vi "统一指令集.vi"(8 "Error In":errorcluster caption="错误输入", 10 "设置参数":string, 11 "统一指令集":T1=enum."波特率切换为9600") -> (0 "Error Out":errorcluster caption="错误输出", 2 "应答":string, 3 "指令":string)   [LabVIEW 2020]
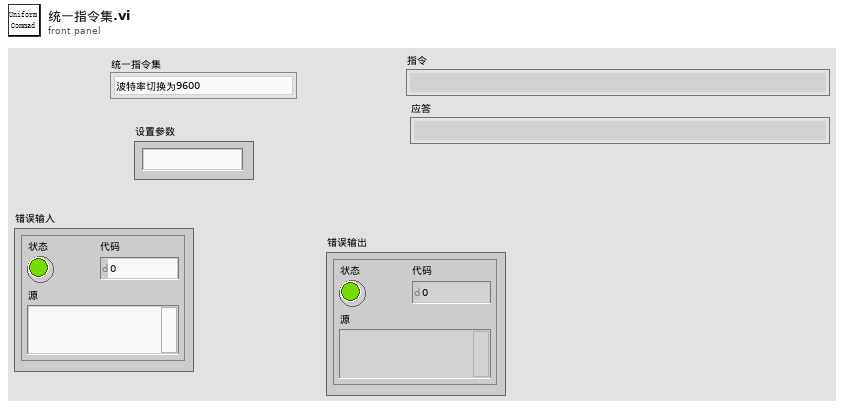
[diagram p1: front panel]
types:
  T1 = typedef "统一指令集.ctl" = enum16{"无操作", "自定义", "波特率切换为9600", "波特率切换为115200", "拍图/解码", "取图", "电平触发模式", "连续读码模式", "睡眠模式", "获取图像分辨率", "开启RTS与CTS流控", "无流控", "感应模式", "红外感应模式", "图像感应模式", "图像与红外感应模式", "切换为串口", "切换为CDC", "关闭照明灯", "开启照明灯", "照明灯常亮", "关闭瞄准灯", "开启瞄准灯", "开启设置码", "连续读码模式2", "触发模式", "0390命令识读模式", "0390连续识读模式", "查询产品序列号", "查询SN空间大小", "产品信息修改开关", "设置产品序列号", "删除序列号", "0390单芯片开启EEPROM写入", "0390单芯片关闭EEPROM写入", "0390单芯片写入产品序列号", "0390单芯片查询产品序列号"}
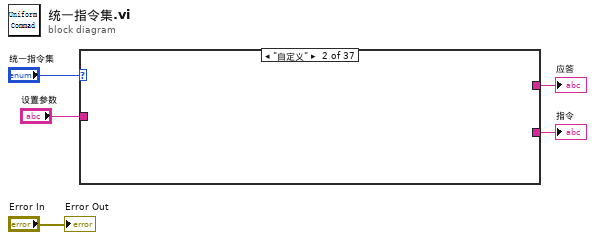
[diagram p0: block diagram]
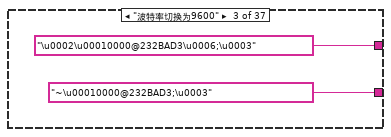
[diagram p3: hidden frame]
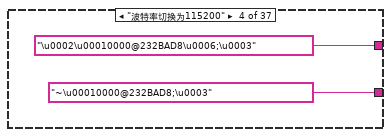
[diagram p4: hidden frame]
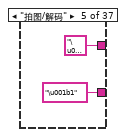
[diagram p5: hidden frame]
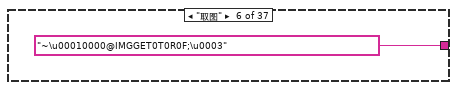
[diagram p6: hidden frame]
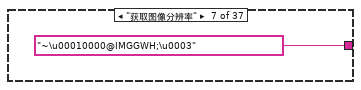
[diagram p7: hidden frame]
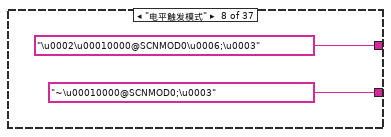
[diagram p8: hidden frame]
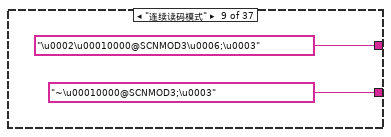
[diagram p9: hidden frame]
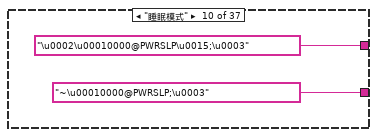
[diagram p10: hidden frame]
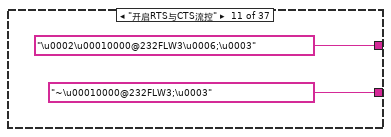
[diagram p11: hidden frame]
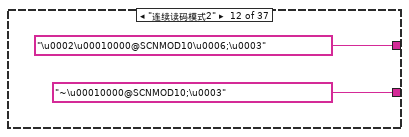
[diagram p12: hidden frame]
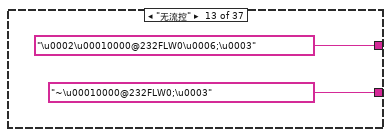
[diagram p13: hidden frame]
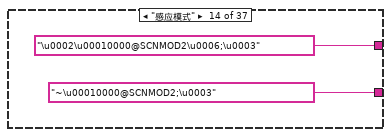
[diagram p14: hidden frame]
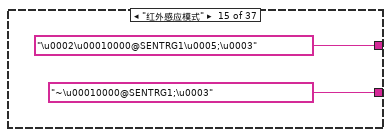
[diagram p15: hidden frame]
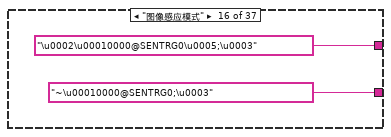
[diagram p16: hidden frame]
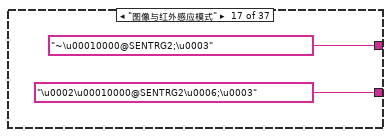
[diagram p17: hidden frame]
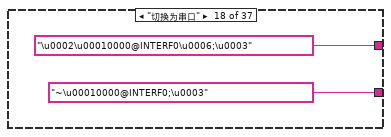
[diagram p18: hidden frame]
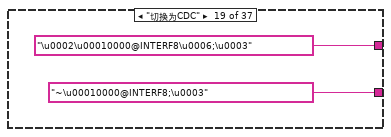
[diagram p19: hidden frame]
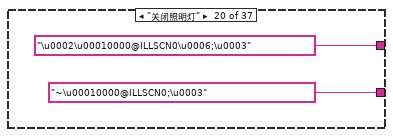
[diagram p20: hidden frame]
diagram:
  n1 = case shown="\"自定义\"" "统一指令集" {
    tunnel: [_ _ "~\u00010000@232BAD3;\u0003" "~\u00010000@232BAD8;\u0003" "\u001b1" "~\u00010000@IMGGET0T0R0F;\u0003" "~\u00010000@IMGGWH;\u0003" "~\u00010000@SCNMOD0;\u0003" "~\u00010000@SCNMOD3;\u0003" "~\u00010000@PWRSLP;\u0003" "~\u00010000@232FLW3;\u0003" "~\u00010000@SCNMOD10;\u0003" "~\u00010000@232FLW0;\u0003" "~\u00010000@SCNMOD2;\u0003" "~\u00010000@SENTRG1;\u0003" "~\u00010000@SENTRG0;\u0003" "\u0002\u00010000@SENTRG2\u0006;\u0003" "~\u00010000@INTERF0;\u0003" "~\u00010000@INTERF8;\u0003" "~\u00010000@ILLSCN0;\u0003" "~\u00010000@ILLSCN1;\u0003" "~\u00010000@ILLSCN2;\u0003" ("设置参数") "~\u00010000@AMLENA0;\u0003" "~\u00010000@AMLENA1;\u0003" "~\u00010000@SETUPN1;\u0003" "~\u00010000@SCNMOD1;\u0003" "~\u0000\b\u0001\u0000\u0000诊\u0004" "~\u0000\b\u0001\u0000\u0000诌\"" "~\u00010000@QRYPSN;\u0003" "~\u00010000@PSNQSZ;\u0003" "~\u00010000@PINFEN1;\u0003" w65 "~\u00010000@PSNDEL;\u0003" "~\u0000\u0003\u0001\u0000\u0000\u0000˜f" "~\u0000\u0000\u0001\u0000\u0000\u0000v´" w74 "~\u0000\u0005\u0001\u0001\u0000\u0000bÓ" ("设置参数")] -> w1
    tunnel: [_ _ "\u0002\u00010000@232BAD3\u0006;\u0003" "\u0002\u00010000@232BAD8\u0006;\u0003" "\u0006" _ _ "\u0002\u00010000@SCNMOD0\u0006;\u0003" "\u0002\u00010000@SCNMOD3\u0006;\u0003" "\u0002\u00010000@PWRSLP\u0015;\u0003" "\u0002\u00010000@232FLW3\u0006;\u0003" "\u0002\u00010000@SCNMOD10\u0006;\u0003" "\u0002\u00010000@232FLW0\u0006;\u0003" "\u0002\u00010000@SCNMOD2\u0006;\u0003" "\u0002\u00010000@SENTRG1\u0005;\u0003" "\u0002\u00010000@SENTRG0\u0005;\u0003" "~\u00010000@SENTRG2;\u0003" "\u0002\u00010000@INTERF0\u0006;\u0003" "\u0002\u00010000@INTERF8\u0006;\u0003" "\u0002\u00010000@ILLSCN0\u0006;\u0003" "\u0002\u00010000@ILLSCN1\u0006;\u0003" "\u0002\u00010000@ILLSCN2\u0006;\u0003" "\u0002\u00010000@AMLENA0\u0006;\u0003" "\u0002\u00010000@AMLENA1\u0006;\u0003" "\u0002\u00010000@SETUPN1\u0006;\u0003" "\u0002\u00010000@SCNMOD1\u0006;\u0003" "\u0002\u0000\u0000\u0001\u000031" "\u0002\u0000\u0000\u0001\u000031" "\r\n\u0006;\u0003" _ "\u0002\u00010000@PINFEN1\u0006;\u0003" w62 "\u0002\u00010000@PSNDEL\u0006;\u0003" "\u0002\u0000\u0000\u0001\u000031" "\u0002\u0000\u0000\u0001\u000031" "\u0002\u0000\u0000\u0001\u000031" _] -> w4
    tunnel: "设置参数" -> [_ _ _ _ _ _ _ _ _ _ _ _ _ _ _ _ _ _ _ _ _ _ _ _ _ _ _ _ _ _ _ w61 _ _ _ w74 _]
    frame "无操作", Default {
    }
    frame "自定义" {
    }
    frame "波特率切换为9600" {
    }
    frame "波特率切换为115200" {
    }
    frame "拍图/解码" {
    }
    frame "取图" {
    }
    frame "获取图像分辨率" {
    }
    frame "电平触发模式" {
    }
    frame "连续读码模式" {
    }
    frame "睡眠模式" {
    }
    frame "开启RTS与CTS流控" {
    }
    frame "连续读码模式2" {
    }
    frame "无流控" {
    }
    frame "感应模式" {
    }
    frame "红外感应模式" {
    }
    frame "图像感应模式" {
    }
    frame "图像与红外感应模式" {
    }
    frame "切换为串口" {
    }
    frame "切换为CDC" {
    }
    frame "关闭照明灯" {
    }
    frame "开启照明灯" {
    }
    frame "照明灯常亮" {
    }
    frame "关闭瞄准灯" {
    }
    frame "开启瞄准灯" {
    }
    frame "开启设置码" {
    }
    frame "触发模式" {
    }
    frame "0390命令识读模式" {
    }
    frame "0390连续识读模式" {
    }
    frame "查询产品序列号" {
    }
    frame "查询SN空间大小" {
    }
    frame "产品信息修改开关" {
    }
    frame "设置产品序列号" {
      n2 = Concatenate Strings("\u0002\u00010000@PSNEDT", w61, "\u0006;\u0003") -> (w62:string)
      n3 = Concatenate Strings("~\u00010000@PSNEDT", w61, ";\u0003") -> (w65:string)
    }
    frame "删除序列号" {
    }
    frame "0390单芯片开启EEPROM写入" {
    }
    frame "0390单芯片关闭EEPROM写入" {
    }
    frame "0390单芯片写入产品序列号" {
    }
    frame "0390单芯片查询产品序列号" {
    }
  }
  "指令" <- w1
  "应答" <- w4
  "Error Out" <- "Error In"
